vi "Sort_Channel_Map.vi"(1 "Channels Map":T1) -> (0 "Sorted Channels Map":T1)   [LabVIEW 2021]
uses:
  Channels_Map.ctl
  Channel_Cluster.ctl
  776d60be-e6e8-4e5a-9e51-e66961cd1bf5.vi
  <vilib>/Comparison/Less/Less Functor/Less Functor.lvclass
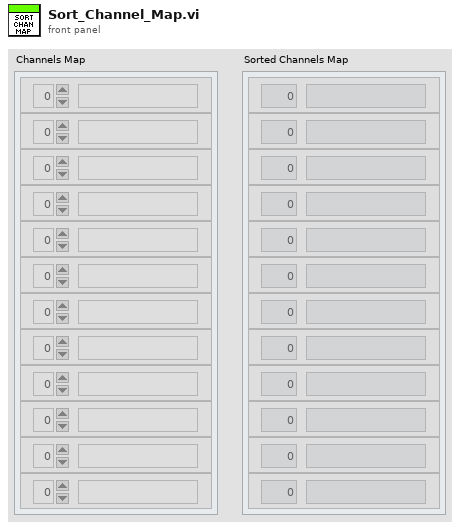
[diagram p1: front panel]
types:
  T1 = typedef "Channels_Map.ctl" = T2[]
  T2 = typedef "Channel_Cluster.ctl" = cluster{"Channel name":string, "Channel":u8}
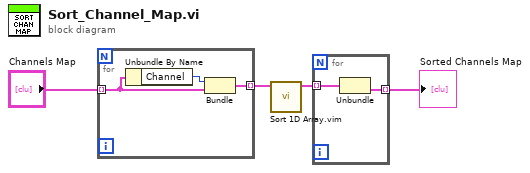
[diagram p0: block diagram]
diagram:
  n1 = for {
    tunnel: "Channels Map" -> [w6] mode=indexing
    tunnel: [w5] -> w4 mode=indexing
    n2 = Unbundle By Name(w6) -> ("Channel"=w7:u8)
    n3 = Bundle("Channel"=w7, "Channel Cluster"=w6) -> (w5:cluster{"Channel":u8, "Channel Cluster":T2})  [unwired: 1 in]
  }
  n4 = call "Sort 1D Array.vim"("unsorted array"=w4) -> ("sorted array"=w3:cluster{"Channel":u8, "Channel Cluster":T2}[])  [unwired: 10 in]
  n5 = for {
    tunnel: w3 -> [w9] mode=indexing
    tunnel: [w8] -> w1 mode=indexing
    n6 = Unbundle(w9) -> ("Channel Cluster"=w8:T2)  [unwired: 1 out]
  }
  "Sorted Channels Map" <- w1
